vi "DWF MSO Read AtoD.vi"(0 "Instrument Handle In AtoD":u32 caption="Instrument Handle In", 11 "Error In":errorcluster caption="Error In (no error)") -> (10 "AtoD":i16, 15 "Error Out":errorcluster)   [LabVIEW 2020]
doc: "Transfers data from the instrument as long as the acquisition state is Acquisition Complete. If the state is either Running or Triggered, this VI will wait until the state transitions to Acquisition Complete. If the state is Stopped, this VI returns an error."
uses:
  dwf.dll
  <vilib>/DigilentWF/DigilentWF.lvlib
panel:
  out "V":dbl
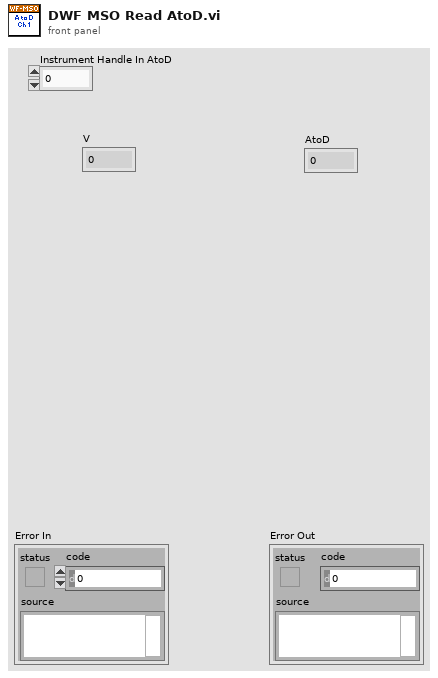
[diagram p1: front panel]
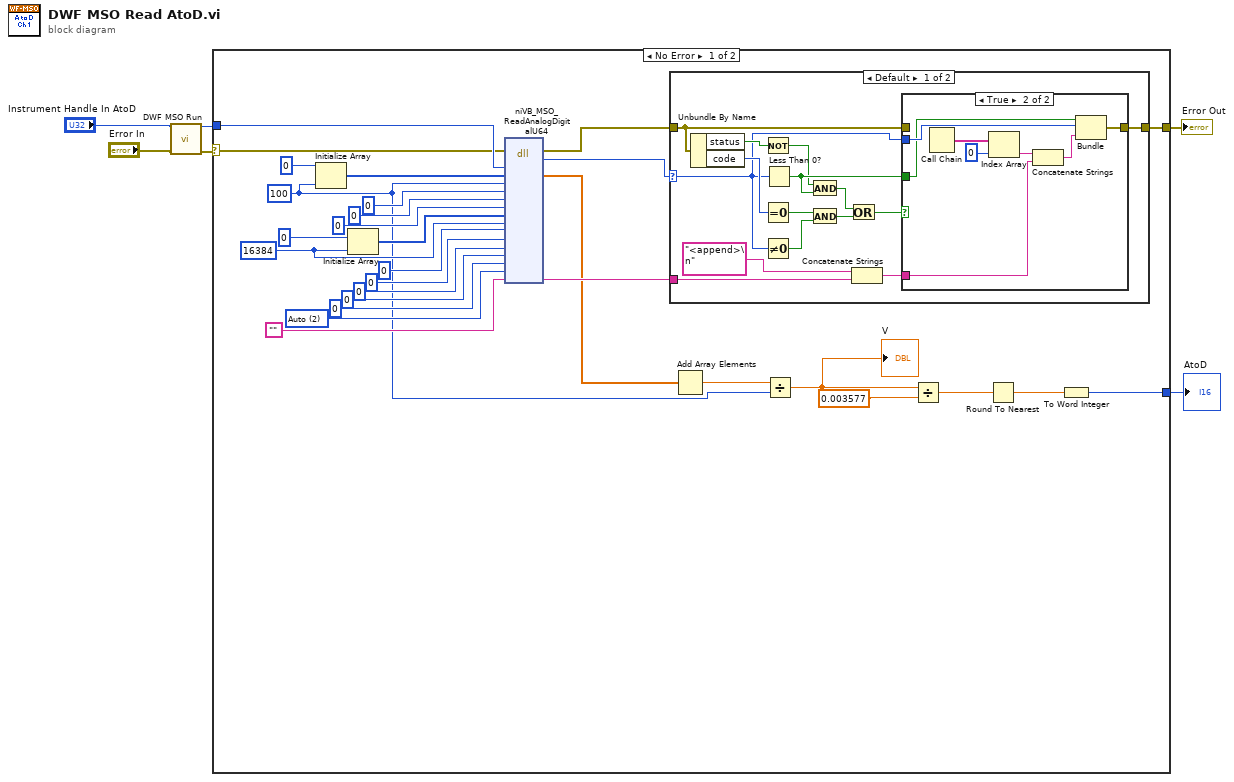
[diagram p0: block diagram]
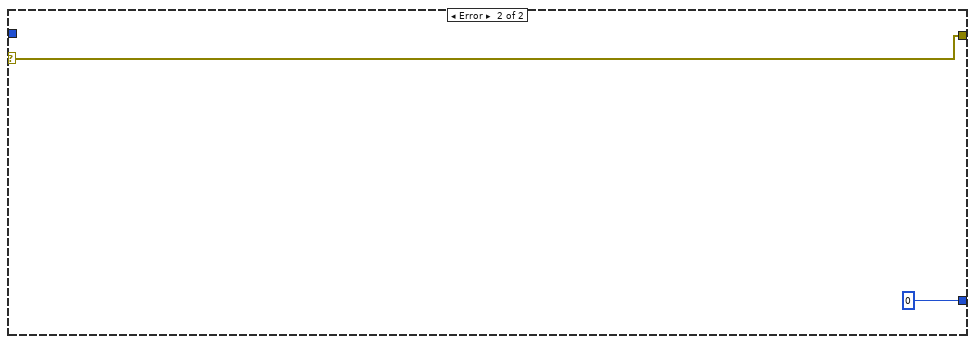
[diagram p4: hidden frame]
diagram:
  n1 = call <vilib>:"DWF MSO Run.vi"("Instrument Handle In"="Instrument Handle In AtoD", "Error In"="Error In") -> ("Instrument Handle Out"=w4:u32, "Error Out"=w3:errorcluster)  [unwired: 12 in]
  n2 = case "outter_case" shown="No Error" w3 {
    selector: w3 -> [w7 w62]
    tunnel: [w35 w62] -> w6
    tunnel: w4 -> [w8 _]
    tunnel: [w11 i16 0] -> w5
    frame No Error {
      w21 = 16384 ("dimension size")
      w9 = 100 ("dimension size")
      w33 = 2 items=["Normal", "Forced", "Auto"] ("Trigger Reason")
      n3 = Initialize Array(0, w9) -> (w24:i32[])
      n4 = Initialize Array(u64 0 ("element"), w21) -> (w22:u64[])
      n5 = dll-call lib="dwf.*" fn="niVB_MSO_ReadAnalogDigitalU64"(error in=w7, "instrumentHandle"=w8, "analogData"=w24, "analogDataSize"=w9, "analogDataSizeOut"=0, "analogDataStride"=0, "analogRate"=0 ("analogInitialTimestamp"), "digitalData"=w22, "digitalDataSize"=w21, "digitalDataSizeOut"=0, "digitalSampleTimestamps"=u32 0, "digitalSampleTimestampsSize"=0, "digitalSampleTimestampsSizeOut"=0, "digitalRate"=0 ("digitalInitialTimestamp"), "triggerReason"=w33, "szError"="") -> (error out=w18:errorcluster, "return type"=w34:i32, "analogData"=w17:dbl[], "szError"=w19:string)  [unwired: 15 in, 1 out]
      n6 = case "inner_case" shown="Default" w34 {
        selector: w34 -> [w40 _]
        tunnel: w18 -> [w41 w60]
        tunnel: [w37 w60] -> w35
        tunnel: w19 -> [w36 _]
        frame Default {
          n7 = Unbundle By Name(w41) -> ("status"=w45:bool, "code"=w49:i32)
          n8 = Not(x=w45) -> (.not. x?=w48:bool)
          n9 = Equal To 0?(x=w49) -> (x = 0?=w44:bool)
          n10 = Not Equal To 0?(x=w40) -> (x != 0?=w47:bool)
          n11 = Less Than 0?(x=w40) -> (x < 0?=w50:bool)
          n12 = And(x=w48, y=w50) -> (x .and. y?=w46:bool)
          n13 = And(x=w44, y=w47) -> (x .and. y?=w43:bool)
          n14 = Or(x=w46, y=w43) -> (x .or. y?=w42:bool)
          n15 = Concatenate Strings("<append>\n" ("string"), w36) -> (w39:string)
          n16 = case shown="True" w42 {
            tunnel: [w51 w58] -> w37
            tunnel: w40 -> [_ w57]
            tunnel: w50 -> [_ w56]
            tunnel: w41 -> [w51 _]
            tunnel: w39 -> [_ w52]
            frame False {
            }
            frame True {
              n17 = Call Chain() -> (call chain=w55:string[])
              n18 = Index Array(array=w55, index=0) -> (element=w54:string)
              n19 = Concatenate Strings(w54, w52) -> (w59:string)
              n20 = Bundle(w56, "return type"=w57, w59) -> (w58:cluster{bool, "return type":i32, string})  [unwired: 1 out]
            }
          }
        }
        frame 0 {
        }
      }
      n21 = Add Array Elements(numeric array=w17) -> (sum=w16:dbl)
      n22 = Divide(x=w16, y=w9) -> (x/y=w13:dbl)
      "V" <- w13
      n23 = Divide(x=w13, y=0.003577) -> (x/y=w14:dbl)
      n24 = Round To Nearest(number=w14) -> (nearest integer value=w12:dbl)
      n25 = To Word Integer(number=w12) -> (16bit integer=w11:i16)
    }
    frame Error {
    }
  }
  "Error Out" <- w6
  "AtoD" <- w5
